vi "Source Settings per Step query.vi"(8 "error in (no error)":errorcluster, 10 "Step":T1=1 min=1 max=99 step=1, 11 "VISA resource name":refnum<visa-resource-name>) -> (0 "error out":errorcluster, 2 "Settings values":string, 3 "VISA resource name out":refnum<visa-resource-name>)   [LabVIEW 2025, in "Chroma 19572.lvlib"]
doc: "Chroma\n5 Clock Tower Place Suite 210\nMaynard, MA 01754\nTel: 1 800 253-1230\nTel: 1 877 4 A HIPOT\nFax: 1 978-461-4295\nWebsite: www.chroma.com"
uses:
  <instrlib>/Chroma 19572/Chroma 19572.lvlib
  <instrlib>/Chroma 19572/Public/Utility/Type Def/steps--numeric.ctl
panel:
  # "Settings values per Step"
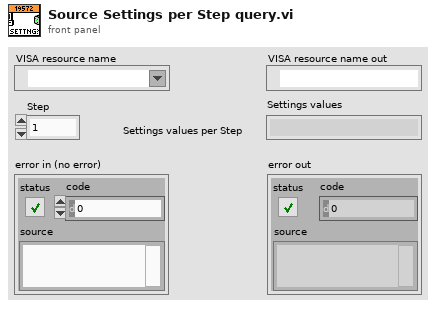
[diagram p1: front panel]
types:
  T1 = typedef "Chroma 19572.lvlib/steps--numeric.ctl" = u8
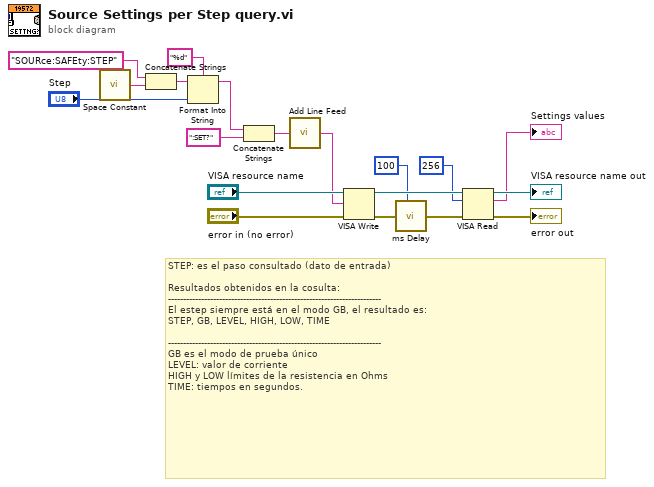
[diagram p0: block diagram]
diagram:
  # "STEP: es el paso consultado (dato de entrada)\n\nResultados obtenidos en la cosulta:\n-----------------------------------------------------------------------\nEl estep siempre está en el modo GB, el resultado es:\nSTEP, GB, LEVEL, HIGH, LOW, TIME\n\n-----------------------------------------------------------------------\nGB es el modo de prueba único\nLEVEL: valor de corriente\nHIGH y LOW límites de la resistencia en Ohms\nTIME: tiempos en segundos."
  n1 = call <vilib>:"Space Constant.vi"() -> ("String"=w5:string)
  n2 = Concatenate Strings("SOURce:SAFEty:STEP", w5) -> (w4:string)
  n3 = Format Into String(format string="%d", initial string=w4, "Step") -> (resulting string=w9:string)  [unwired: 1 in, 1 out]
  n4 = Concatenate Strings(w9, ":SET?") -> (w7:string)
  n5 = call <instrlib>:"Add Line Feed.vi"("Command string"=w7) -> ("Concatenated string"=w15:string)  [unwired: 4 in]
  n6 = VISA Write(VISA resource name="VISA resource name", write buffer=w15, error in (no error)="error in (no error)") -> (VISA resource name out=w19:refnum<visa-resource-name>, error out=w3:errorcluster)  [unwired: 1 out]
  n7 = call <instrlib>:"ms Delay.vi"("miliseconds to wait"=u32 100 ("Time Delay ms"), "error in (no error)"=w3) -> ("error out"=w2:errorcluster)  [unwired: 6 in, 1 out]
  n8 = VISA Read(VISA resource name=w19, byte count=u32 256, error in (no error)=w2) -> (VISA resource name out=→"VISA resource name out":refnum<visa-resource-name>, read buffer=→"Settings values":string, error out=→"error out":errorcluster)  [unwired: 1 out]
